vi "update running sums.vi"(8 "current location":T1, 9 "integration channels":enum16{"channel 0", "channel 1", "both"}(ring), 10 "sampling values in":T3, 11 "running sums in":T2) -> (3 "running sums out":T2)   [LabVIEW 2010]
uses:
  common_typedefs/channels_cluster.ctl
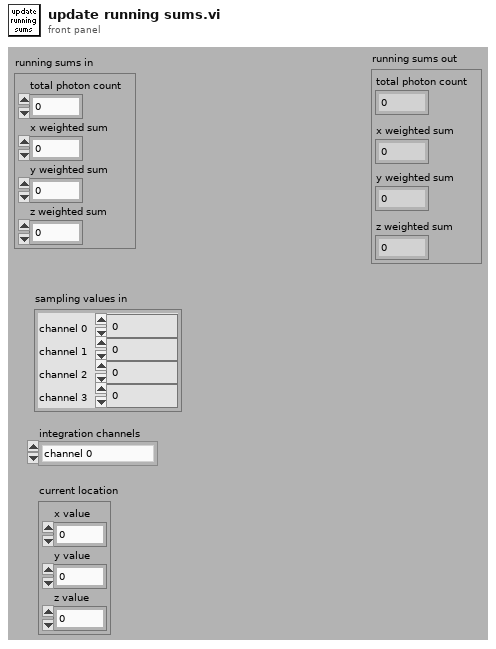
[diagram p1: front panel]
types:
  T1 = cluster{"x value":i16, "y value":i16, "z value":i16}
  T2 = cluster{"total photon count":u32, "x weighted sum":i32, "y weighted sum":i32, "z weighted sum":i32}
  T3 = typedef "channels_cluster.ctl" = cluster{"channel 0":u32, "channel 1":u32, "channel 2":u32, "channel 3":u32}
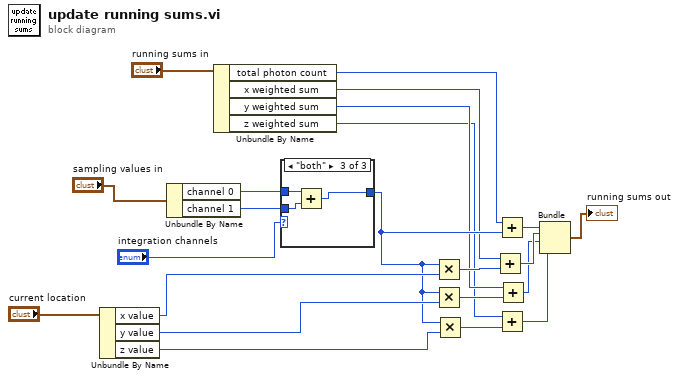
[diagram p0: block diagram]
diagram:
  n1 = Unbundle By Name("current location") -> ("x value"=w16:i16, "y value"=w15:i16, "z value"=w14:i16)
  n2 = Unbundle By Name("sampling values in") -> ("channel 0"=w20:u32, "channel 1"=w19:u32)
  n3 = Unbundle By Name("running sums in") -> ("total photon count"=w9:u32, "x weighted sum"=w8:i32, "y weighted sum"=w7:i32, "z weighted sum"=w6:i32)
  n4 = case shown="\"both\"" "integration channels" {
    tunnel: [w23 w24 w25] -> w10
    tunnel: w20 -> [w23 _ w27]
    tunnel: w19 -> [_ w24 w26]
    frame "channel 0", Default {
    }
    frame "channel 1" {
    }
    frame "both" {
      n5 = Add(x=w27, y=w26) -> (x+y=w25:u32)
    }
  }
  n6 = Multiply(x=w10, y=w16) -> (x*y=w13:i32)
  n7 = Multiply(x=w10, y=w15) -> (x*y=w12:i32)
  n8 = Multiply(x=w10, y=w14) -> (x*y=w11:i32)
  n9 = Add(x=w8, y=w13) -> (x+y=w4:i32)
  n10 = Add(x=w9, y=w10) -> (x+y=w5:u32)
  n11 = Add(x=w6, y=w11) -> (x+y=w2:i32)
  n12 = Add(x=w7, y=w12) -> (x+y=w3:i32)
  n13 = Bundle(w5, w4, w3, w2) -> (→"running sums out":cluster{u32, i32, i32, i32})  [unwired: 1 in]
